vi "Rotation3d_Minus.vi"(9 "other Rotation3d":T1={"Q_quaternion"={"R"=1.0, "V"=[0.0, 0.0, 0.0]}}, 11 "in Rotation3d":T1={"Q_quaternion"={"R"=1.0, "V"=[0.0, 0.0, 0.0]}}) -> (3 "out Rotation3d":T1={"Q_quaternion"={"R"=1.0, "V"=[0.0, 0.0, 0.0]}})   [LabVIEW 2019, in "Trajectory_Library.lvlib"]
doc: "Subtracts the new rotation from the current rotation and returns the new rotation.\n\nFor example, Rotation2d.fromDegrees(10) - Rotation2d.fromDegrees(100) = Rotation2d{-pi/2}\n\nParameters:\n- in ROTATION - This rotation data structure\n - other ROTATION - The rotation to subtract.\n\nReturns:\n - out ROTATION - The difference between the two rotations."
uses:
  Trajectory_Library.lvlib
  ROTATION3D.ctl
  QUATERNION.ctl
  Rotation3d_Create_Quaternion.vi
  Quaternion_Inverse.vi
  Rotation3d_GetQuaterion.vi
  Quaternion_Times.vi
  Quaternion_Normalize.vi
  Quaternion_New_Default.vi
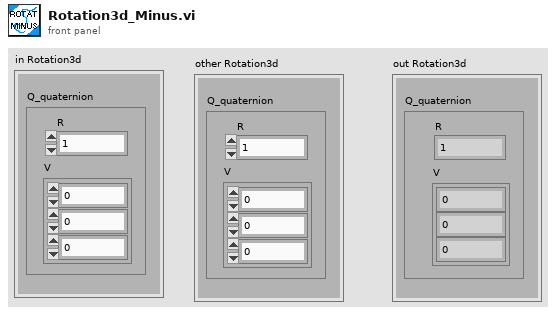
[diagram p1: front panel]
types:
  T1 = typedef "Trajectory_Library.lvlib/ROTATION3D.ctl" = cluster{"Q_quaternion":T2}
  T2 = typedef "Trajectory_Library.lvlib/QUATERNION.ctl" = cluster{"R":dbl, "V":dbl[]}
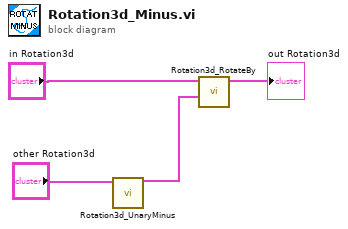
[diagram p0: block diagram]
diagram:
  n1 = call "Rotation3d_UnaryMinus.vi"("in Rotation3d"="other Rotation3d") -> ("out Rotation3d"=w1:T1)  [unwired: 10 in]
  n2 = call "Rotation3d_RotateBy.vi"("other Rotation3d"=w1, "in Rotation3d"="in Rotation3d") -> ("out Rotation3d"=→"out Rotation3d":T1)  [unwired: 9 in]
